vi "CreateTransaction.vi"(7 "error in (no error)":errorcluster, 8 "BN":string, 9 "SN":string, 10 "reference in":refnum<class "MES_Local.lvclass">) -> (0 "error out":errorcluster, 1 "OK":bool, 3 "reference in":refnum<class "MES_Local.lvclass">)   [LabVIEW 2022 SP3, in "MES_Local.lvlib" / "MES_Local.lvclass"]
uses:
  MES_Local.lvclass
  Components/MES_Base.lvlibp/MES_Base.lvclass
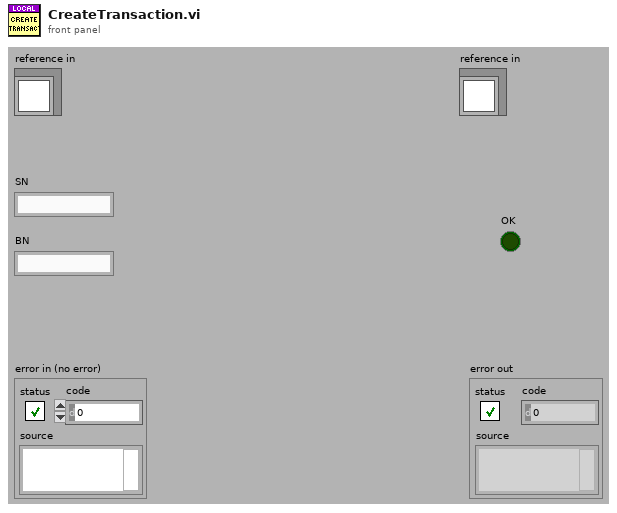
[diagram p1: front panel]
types:
  T1 = typedef "MES_Local.lvlib/MES_Local.lvclass/ObjectAttributes.ctl" = cluster{"Config":T2, "Logged_In?":bool, "AttributeNames":string[], "AttributeWritten":bool[], "ComponentNames":string[], "TestIndex":i32, "TestTag":string[], "Time Stamp":timestamp, "Employee":string, "Resource_Key":string, "Local Spec":path, "Login":refnum<class "Login_Base.lvclass">, "ReportPath":path, "Spec":T3, "StartTime":timestamp, "Role":string}
  T2 = typedef "MES_Local.lvlib/MES_Local.lvclass/Config.ctl" = cluster{"Results_Path":path}
  T3 = typedef "MES_Base.lvlibp/MES_Base.lvclass/Spec.ctl" = cluster{"Header":cluster{"Doctype":string, "Checksum":string, "DriverKey":string, "SpecId":string, "TransactionId":string, "AccountId":string, "SpecName":string, "WorkflowStep":string, "SerialNumber":string, "BatchNumber":string, "Status":enum16{"Pending", "Pass", "Fail"}, "Comment":string, "FirstFail":string, "Employee":string, "LocalMachine":string, "ResourceKey":string, "Date":string, "Time":string, "Duration":string, "DUT Position":i32}, "Components":cluster{"SerialNumber":string, "PartNumber":string, "Revision":string, "BatchNumber":string, "Name":string, "Description":string, "Attached":bool}[], "Attributes":cluster{"Name":string, "Description":string, "DataType":enum16{"NA", "String", "Boolean", "Int", "Dbl"}, "Value":variant, "DisplayFormat":string, "ReadOnly":bool, "Required":bool}[], "Tests":cluster{"Code":string, "Name":string, "Description":string, "Group":string, "IsGroup":bool, "Tag":string, "Method":string, "Parrameter":string, "DataType":enum16{"NA", "String", "Boolean", "Int", "Dbl"}, "Value":variant, "Status":enum16{"Pending", "Pass", "Fail"}, "LimitLo":variant, "LimitHi":variant, "StringMatch":string, "BooleanMatch":bool, "DisplayFormat":string, "Units":string, "TestTime":dbl}[]}
  T4 = cluster{"Header":cluster{"Doctype":string, "Checksum":string, "DriverKey":string, "SpecId":string, "TransactionId":string, "AccountId":string, "SpecName":string, "WorkflowStep":string, "SerialNumber":string, "BatchNumber":string, "Status":enum16{"Pending", "Pass", "Fail"}, "Comment":string, "FirstFail":string, "Employee":string, "LocalMachine":string, "ResourceKey":string, "Date":string, "Time":string, "Duration":string, "DUT Position":i32}, "Components":cluster{"SerialNumber":string, "PartNumber":string, "Revision":string, "BatchNumber":string, "Name":string, "Description":string, "Attached":bool}[], "Attributes":cluster{"Name":string, "Description":string, "DataType":enum16{"NA", "String", "Boolean", "Int", "Dbl"}, "Value":variant, "DisplayFormat":string, "ReadOnly":bool, "Required":bool}[], "Tests":cluster{"Code":string, "Name":string, "Description":string, "Group":string, "IsGroup":bool, "Tag":string, "Method":string, "Parrameter":string, "DataType":enum16{"NA", "String", "Boolean", "Int", "Dbl"}, "Value":variant, "Status":enum16{"Pending", "Pass", "Fail"}, "LimitLo":variant, "LimitHi":variant, "StringMatch":string, "BooleanMatch":bool, "DisplayFormat":string, "Units":string, "TestTime":dbl}[]}
  T5 = cluster{"Name":string, "Description":string, "DataType":enum16{"NA", "String", "Boolean", "Int", "Dbl"}, "Value":variant, "DisplayFormat":string, "ReadOnly":bool, "Required":bool}[]
  T6 = cluster{"SerialNumber":string, "PartNumber":string, "Revision":string, "BatchNumber":string, "Name":string, "Description":string, "Attached":bool}[]
  T7 = cluster{"Code":string, "Name":string, "Description":string, "Group":string, "IsGroup":bool, "Tag":string, "Method":string, "Parrameter":string, "DataType":enum16{"NA", "String", "Boolean", "Int", "Dbl"}, "Value":variant, "Status":enum16{"Pending", "Pass", "Fail"}, "LimitLo":variant, "LimitHi":variant, "StringMatch":string, "BooleanMatch":bool, "DisplayFormat":string, "Units":string, "TestTime":dbl}[]
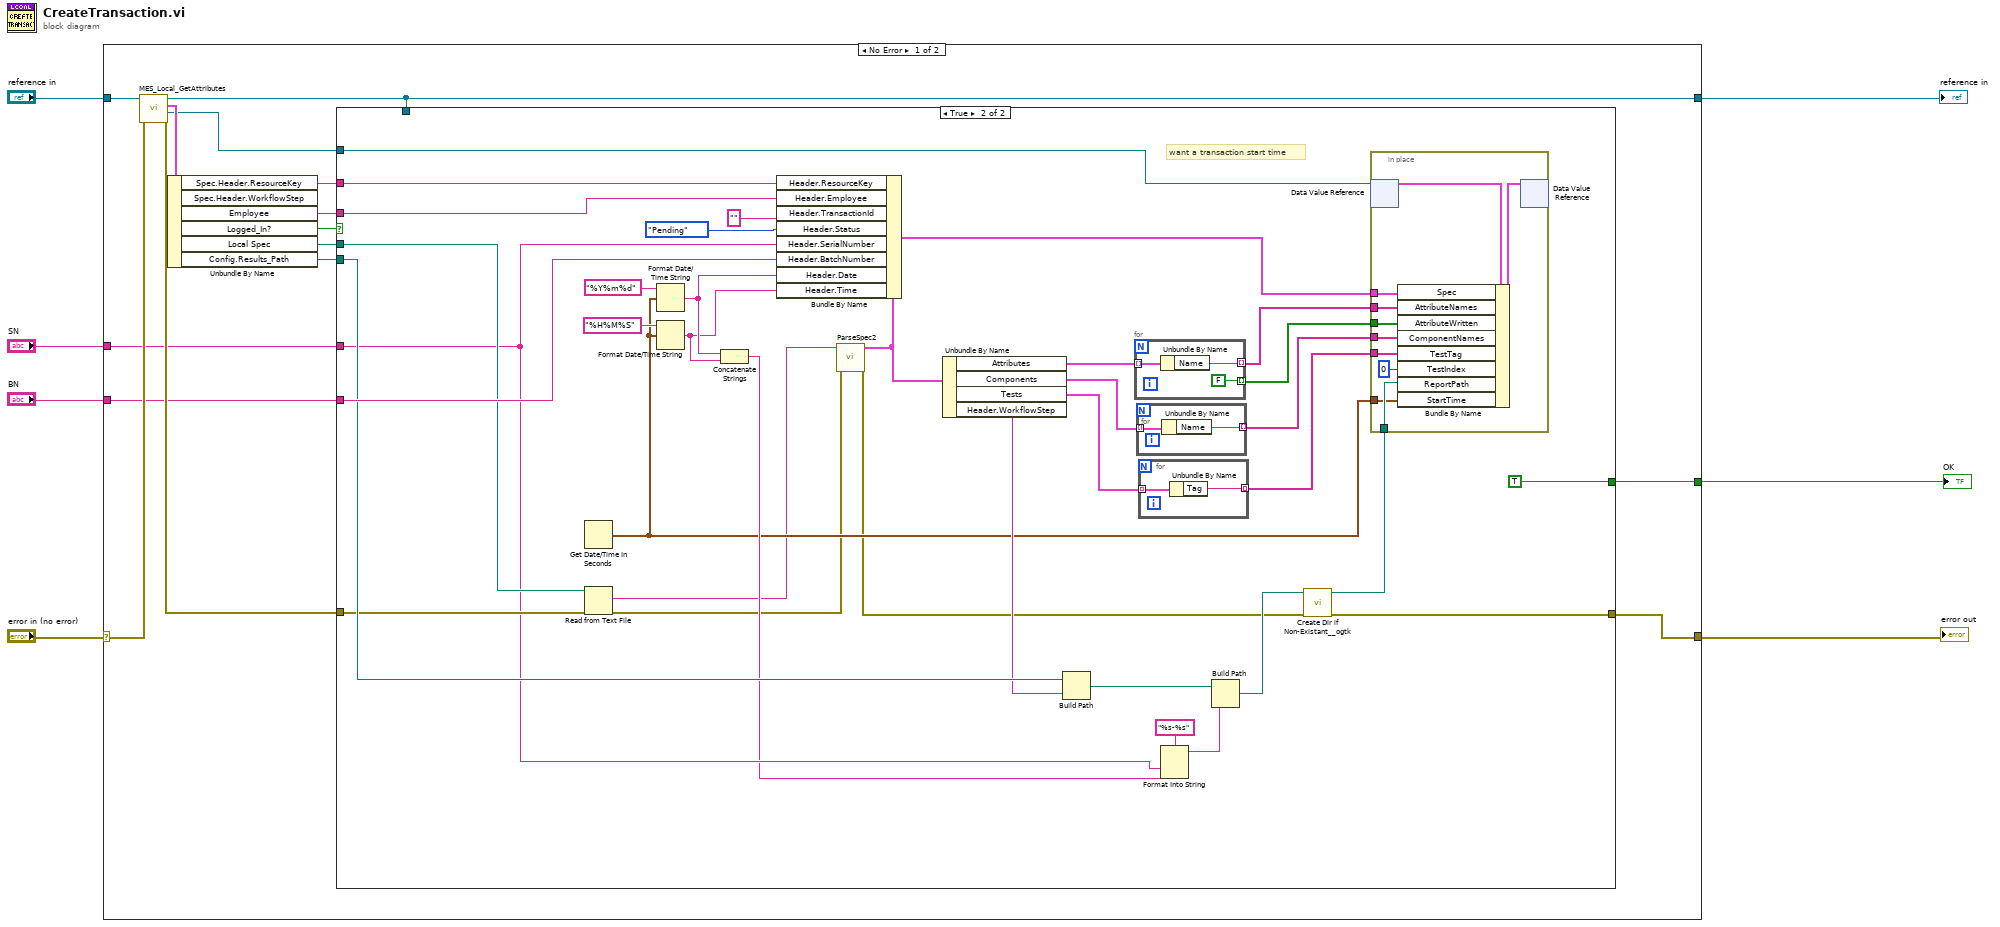
[diagram p0: block diagram]
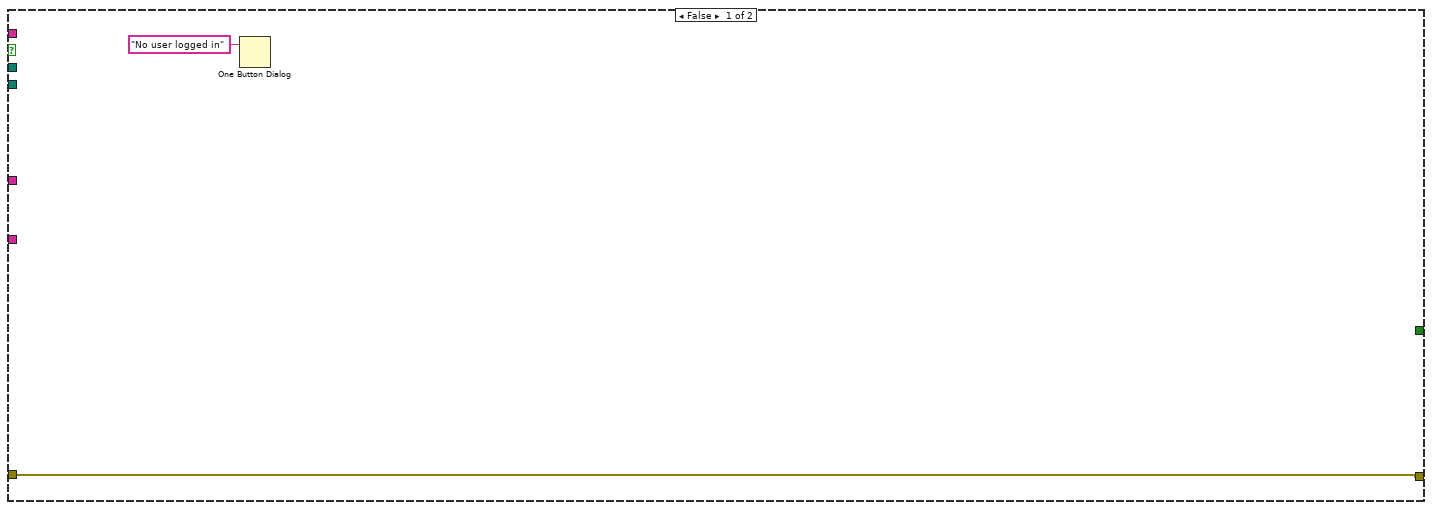
[diagram p2: hidden frame]
diagram:
  n1 = case shown="No Error" "error in (no error)" {
    selector: "error in (no error)" -> [w22 w79]
    tunnel: [w17 w79] -> w6
    tunnel: [w9 w78] -> w4
    tunnel: "reference in" -> [w20 w78]
    tunnel: "BN" -> [w16 _]
    tunnel: "SN" -> [w15 _]
    tunnel: [w11 _] -> w1
    frame No Error {
      n2 = call "MES_Local_GetAttributes.vi"("error in (no error)"=w22, "reference in"=w20) -> ("error out"=w18:errorcluster, "DataRef"=w14:refnum<data-value>, "Data"=w21:T1, "reference out"=w9:refnum<class "MES_Local.lvclass">)  [unwired: 6 in]
      n3 = Unbundle By Name(w21) -> ("Spec.Header.ResourceKey"=w12:string, "Employee"=w13:string, "Logged_In?"=w19:bool, "Local Spec"=w10:path, "Config.Results_Path"=w8:path)  [unwired: 1 out]
      n4 = case shown="True" w19 {
        tunnel: w18 -> [w24 w39]
        tunnel: [w24 w33] -> w17
        tunnel: w16 -> [_ w60]
        tunnel: w15 -> [_ w36]
        tunnel: w14 -> [_ w59]
        tunnel: w13 -> [_ w58]
        tunnel: w12 -> [_ w57]
        tunnel: [_ TRUE] -> w11
        tunnel: w10 -> [_ w43]
        tunnel: w9 -> [_ _]
        tunnel: w8 -> [_ w40]
        frame False {
          n5 = One Button Dialog(message="No user logged in") -> ()  [unwired: 1 in, 1 out]
        }
        frame True {
          # "want a transaction start time"
          n6 = Get Date/Time In Seconds() -> (seconds since 1Jan1904=w29:timestamp)
          n7 = Read from Text File(file (use dialog)=w43, error in=w39) -> (text=w28:string, error out=w26:errorcluster)  [unwired: 2 in, 2 out]
          n8 = Format Date/Time String(time format string (%c)="%Y%m%d", seconds (now)=w29) -> (date/time string=w32:string)  [unwired: 1 in]
          n9 = Format Date/Time String(time format string (%c)="%H%M%S", seconds (now)=w29) -> (date/time string=w31:string)  [unwired: 1 in]
          n10 = Concatenate Strings(w32, w31) -> (w30:string)
          n11 = call "ParseSpec2.vi"("error in (no error)"=w26, "Spec XML"=w28) -> ("error out"=w25:errorcluster, "Spec"=w27:T4)  [unwired: 8 in]
          n12 = Bundle By Name(cluster=w27, "Header.ResourceKey"=w57, "Header.Employee"=w58, "Header.TransactionId"="", "Header.Status"=enum16{"Pending", "Pass", "Fail"}."Pending", "Header.SerialNumber"=w36, "Header.BatchNumber"=w60, "Header.Date"=w32, "Header.Time"=w31) -> (w48:T4)
          n13 = Unbundle By Name(w27) -> ("Attributes"=w53:T5, "Components"=w54:T6, "Tests"=w55:T7, "Header.WorkflowStep"=w38:string)
          n14 = Build Path(base path=w40, name or relative path=w38) -> (appended path=w41:path)
          n15 = for {
            tunnel: w53 -> [w77] mode=indexing
            tunnel: [w76] -> w52 mode=indexing
            tunnel: [FALSE] -> w51 mode=indexing
            n16 = Unbundle By Name(w77) -> ("Name"=w76:string)
          }
          n17 = for {
            tunnel: w54 -> [w74] mode=indexing
            tunnel: [w73] -> w50 mode=indexing
            n18 = Unbundle By Name(w74) -> ("Name"=w73:string)
          }
          n19 = for {
            tunnel: w55 -> [w72] mode=indexing
            tunnel: [w71] -> w49 mode=indexing
            n20 = Unbundle By Name(w72) -> ("Tag"=w71:string)
          }
          n21 = Format Into String(format string="%s-%s", w36, w30) -> (resulting string=w35:string)  [unwired: 2 in, 1 out]
          n22 = Build Path(base path=w41, name or relative path=w35) -> (appended path=w42:path)
          n23 = call <userlib>:"Create Dir if Non-Existant__ogtk.vi"("error in (no error)"=w25, "Directory Path"=w42) -> ("error out"=w33:errorcluster, "dup Directory Path"=w34:path)  [unwired: 7 in, 1 out]
          n24 = in-place {
            in-place-border: w52 -> [w68]
            in-place-border: w51 -> [w67]
            in-place-border: w50 -> [w66]
            in-place-border: w49 -> [w65]
            in-place-border: w48 -> [w64]
            in-place-border: w34 -> [w62]
            in-place-border: w29 -> [w61]
            n25 = in-place-dvr #1(w59) -> (w70:T1)  [unwired: 1 out]
            n26 = Bundle By Name(cluster=w70, "Spec"=w64, "AttributeNames"=w68, "AttributeWritten"=w67, "ComponentNames"=w66, "TestTag"=w65, "TestIndex"=0, "ReportPath"=w62, "StartTime"=w61) -> (w69:T1)
            n27 = in-place-dvr #1(w69) -> ()  [unwired: 2 out]
          }
        }
      }
    }
    frame Error {
    }
  }
  "error out" <- w6
  "reference in" <- w4
  "OK" <- w1
